vi "colortest2.vi"() -> ()   [LabVIEW 2018]
panel:
  in  "动态显示选择":enum16{"最高点6dB范围", "固定范围", "手动选择", "手动选择？"}(ring)
  in  "System Link Text 2":bool
  in  "System Link Text":bool
  out "H 7":T1(plugin-control)
  in  "停止":bool
  in  "dB最大值":dbl=50.0
  in  "显示dB长度":dbl=50.0
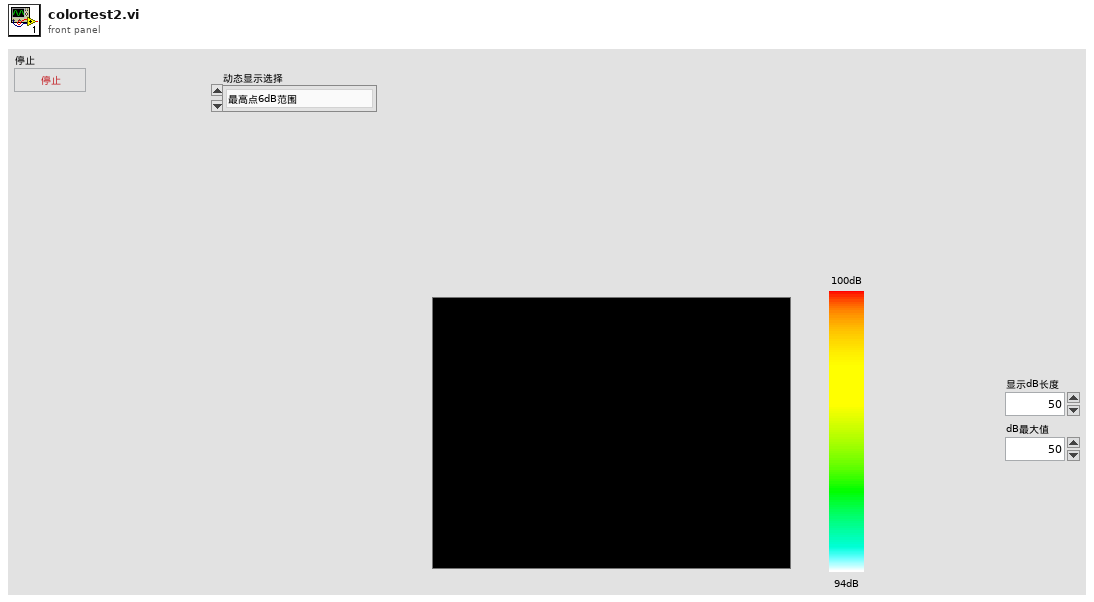
[diagram p1: front panel]
types:
  T1 = typedef "IMAQ Image.ctl" = refnum<image>
  T2 = typedef "Image Type" = u32
  T3 = cluster{"Image Out":T1, "Image Out":T1, "Image Out":T1, "Image Out":T1, "Image Out":T1}
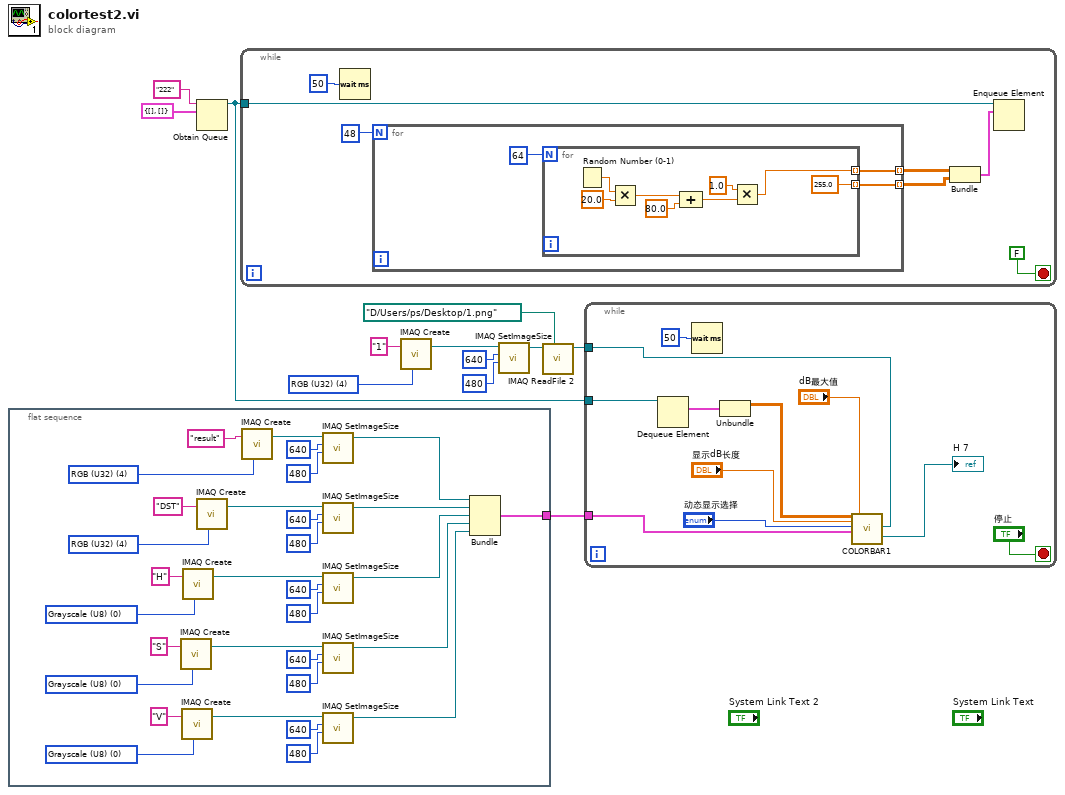
[diagram p0: block diagram]
diagram:
  w10 = T2 4 items=["Grayscale (U8)", "Grayscale (I16)", "Grayscale (SGL)", "Complex (CSG)", "RGB (U32)", "HSL (U32)", "RGB (U64)", "Grayscale (U16)"] ("Image Type")
  n1 = flat-sequence {
    tunnel: [w13] -> w1
    frame #0 {
      w21 = T2 4 items=["Grayscale (U8)", "Grayscale (I16)", "Grayscale (SGL)", "Complex (CSG)", "RGB (U32)", "HSL (U32)", "RGB (U64)", "Grayscale (U16)"] ("Image Type")
      w26 = T2 4 items=["Grayscale (U8)", "Grayscale (I16)", "Grayscale (SGL)", "Complex (CSG)", "RGB (U32)", "HSL (U32)", "RGB (U64)", "Grayscale (U16)"] ("Image Type")
      w31 = T2 0 items=["Grayscale (U8)", "Grayscale (I16)", "Grayscale (SGL)", "Complex (CSG)", "RGB (U32)", "HSL (U32)", "RGB (U64)", "Grayscale (U16)"] ("Image Type")
      w36 = T2 0 items=["Grayscale (U8)", "Grayscale (I16)", "Grayscale (SGL)", "Complex (CSG)", "RGB (U32)", "HSL (U32)", "RGB (U64)", "Grayscale (U16)"] ("Image Type")
      w41 = T2 0 items=["Grayscale (U8)", "Grayscale (I16)", "Grayscale (SGL)", "Complex (CSG)", "RGB (U32)", "HSL (U32)", "RGB (U64)", "Grayscale (U16)"] ("Image Type")
      n2 = call "IMAQ Create"("Image Name"="S", "Image Type"=w36) -> ("New Image"=w38:T1)  [unwired: 3 in, 1 out]
      n3 = call "IMAQ Create"("Image Name"="V", "Image Type"=w31) -> ("New Image"=w33:T1)  [unwired: 3 in, 1 out]
      n4 = call "IMAQ Create"("Image Name"="H", "Image Type"=w41) -> ("New Image"=w43:T1)  [unwired: 3 in, 1 out]
      n5 = call "IMAQ Create"("Image Name"="DST", "Image Type"=w26) -> ("New Image"=w28:T1)  [unwired: 3 in, 1 out]
      n6 = call "IMAQ Create"("Image Name"="result", "Image Type"=w21) -> ("New Image"=w23:T1)  [unwired: 3 in, 1 out]
      n7 = call "IMAQ SetImageSize"("Y Resolution"=480, "X Resolution"=640, "Image"=w23) -> ("Image Out"=w14:T1)  [unwired: 2 in, 1 out]
      n8 = call "IMAQ SetImageSize"("Y Resolution"=480, "X Resolution"=640, "Image"=w28) -> ("Image Out"=w15:T1)  [unwired: 2 in, 1 out]
      n9 = call "IMAQ SetImageSize"("Y Resolution"=480, "X Resolution"=640, "Image"=w43) -> ("Image Out"=w16:T1)  [unwired: 2 in, 1 out]
      n10 = call "IMAQ SetImageSize"("Y Resolution"=480, "X Resolution"=640, "Image"=w38) -> ("Image Out"=w17:T1)  [unwired: 2 in, 1 out]
      n11 = call "IMAQ SetImageSize"("Y Resolution"=480, "X Resolution"=640, "Image"=w33) -> ("Image Out"=w18:T1)  [unwired: 2 in, 1 out]
      n12 = Bundle("Image Out"=w14, "Image Out"=w15, "Image Out"=w16, "Image Out"=w17, "Image Out"=w18) -> (w13:T3)  [unwired: 1 in]
    }
  }
  n13 = Obtain Queue(name (unnamed)="222" ("名称（未命名）"), element data type=cluster{dbl[][], dbl[][]} {[], []} ("输出簇")) -> (queue out=w2:refnum<queue>)  [unwired: 3 in, 2 out]
  n14 = while {
    tunnel: w2 -> [w47]
    stop <- FALSE stop-if-true
    n15 = Wait (ms)(milliseconds to wait=u32 50 ("等待时间（毫秒）")) -> ()  [unwired: 1 out]
    n16 = for {
      N: 48 -> [_]
      tunnel: [w53] -> w44 mode=indexing
      tunnel: [w51] -> w49 mode=indexing
      n17 = for {
        N: 64 -> [_]
        tunnel: [w56] -> w53 mode=indexing
        tunnel: [255.0] -> w51 mode=indexing
        n18 = Random Number (0-1)() -> (number: 0 to 1=w59:dbl)
        n19 = Multiply(x=w59, y=20.0 ("x")) -> (x*y=w58:dbl)
        n20 = Compound Arithmetic op=ADD(w58, 80.0 ("值")) -> (w57:dbl)
        n21 = Multiply(x=1.0, y=w57) -> (x*y=w56:dbl)
      }
    }
    n22 = Bundle(w44, w49) -> (w48:cluster{dbl[][], dbl[][]})  [unwired: 1 in]
    n23 = Enqueue Element(queue=w47, element=w48) -> ()  [unwired: 2 in, 3 out]
  }
  n24 = call "IMAQ Create"("Image Name"="1", "Image Type"=w10) -> ("New Image"=w12:T1)  [unwired: 3 in, 1 out]
  n25 = call "IMAQ SetImageSize"("Y Resolution"=480, "X Resolution"=640, "Image"=w12) -> ("Image Out"=w7:T1)  [unwired: 2 in, 1 out]
  n26 = call "IMAQ ReadFile 2"("File Path"=path "D:/Users/ps/Desktop/1.png", "Image"=w7) -> ("Image Out"=w5:T1)  [unwired: 5 in, 4 out]
  n27 = while {
    tunnel: w2 -> [w71]
    tunnel: w1 -> [w64]
    tunnel: w5 -> [w63]
    stop <- "停止" stop-if-true
    n28 = Dequeue Element(queue=w71) -> (element=w70:cluster{dbl[][], dbl[][]})  [unwired: 2 in, 3 out]
    n29 = Wait (ms)(milliseconds to wait=u32 50 ("等待时间（毫秒）")) -> ()  [unwired: 1 out]
    n30 = Unbundle(w70) -> (w67:dbl[][])  [unwired: 1 out]
    n31 = call "COLORBAR1.vi"("数组"=w67, "显示dB长度"="显示dB长度", "动态显示选择"="动态显示选择", "簇"=w64, "dB最大值"="dB最大值", "Image Out"=w63) -> ("H 7"=→"H 7":T1)  [unwired: 11 in, 2 out]
  }
